vi "TWM Client Cmd Get Versions.vi"(5 "timeout [ms] (3000)":i32=3000, 7 "end of packet key":string="TWM:command:EndOfPacket", 8 "error in":errorcluster, 11 "handle":i32) -> (0 "error out":errorcluster, 2 "TWM client version string":string, 3 "handle out":i32)   [LabVIEW 2020, in "TWM Client.lvlib"]
doc: "Retrieves version of TWM client and TWM itself."
uses:
  TWM Client.lvlib
  GetString.vi
  <vilib>/Utility/error.llb/Error Cluster From Error Code.vi
  <vilib>/ErrorRing/Error Ring.xnode
  infolib.lvlib
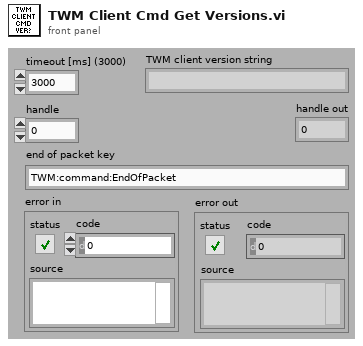
[diagram p1: front panel]
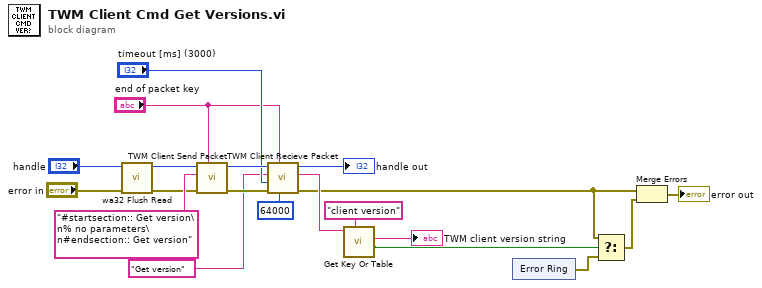
[diagram p0: block diagram]
diagram:
  n1 = call "wa32 Flush Read.vi"("error in"="error in", "handle"="handle") -> ("error out"=w3:errorcluster, "handle out"=w2:i32)  [unwired: 7 in, 1 out]
  n2 = call "TWM Client Send Packet.vi"("end of packet key"="end of packet key", "error in"=w3, "command string"="#startsection:: Get version\n% no parameters\n#endsection:: Get version", "handle"=w2) -> ("error out"=w17:errorcluster, "handle out"=w15:i32)  [unwired: 6 in]
  n3 = call "TWM Client Recieve Packet.vi"("max message length (1024)"=64000, "end of packet key"="end of packet key", "error in"=w17, "timeout [ms] (5000 ms)"="timeout [ms] (3000)", "message header (empty)"="Get version" ("key string"), "handle in"=w15) -> ("error out"=w8:errorcluster, "message data"=w10:string, "handle out"=→"handle out":i32)  [unwired: 3 in]
  n4 = call-poly "Get Key Or Table.vi"("key description"="client version", "info data"=w10) -> ("key found?"=w5:bool, "value"=→"TWM client version string":string)  [unwired: 6 in, 2 out]
  n5 = xnode "Error Ring"() -> ("error out"=w9:errorcluster)
  n6 = Select(t=w8, s=w5, f=w9) -> (s? t:f=w7:errorcluster)
  n7 = Merge Errors(w8, w7) -> (→"error out":errorcluster)
